vi "Add Alias_Alias.vi"(8 "error in (no error)":errorcluster, 10 "Alias Settings":T1, 11 "Aliases Ref":refnum<k24>) -> (0 "error out":errorcluster, 3 "Aliases Ref Out":refnum<k24>)   [LabVIEW 2019, in "Simple SysDef API.lvlib"]
uses:
  <userlib>/SimpleSysDef/Simple SysDef API.lvlib
  NationalInstruments.VeriStand.SystemDefinitionAPI
  <userlib>/SimpleSysDef/_SubVIs/Add Alias_Alias Settings.ctl
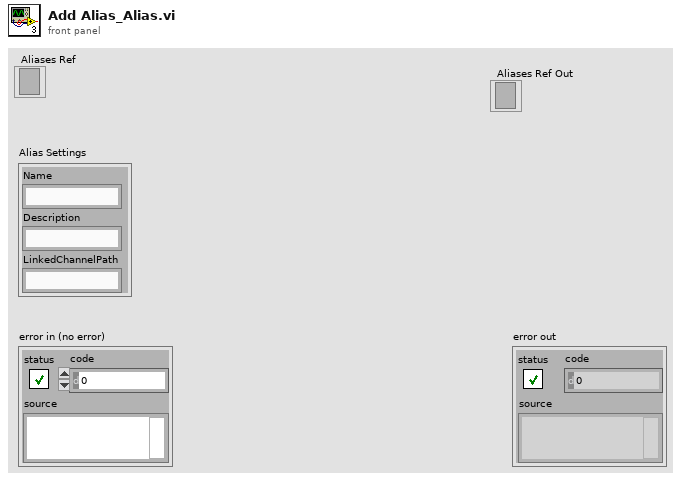
[diagram p1: front panel]
types:
  T1 = typedef "Simple SysDef API.lvlib/Add Alias_Alias Settings.ctl" = cluster{"Name":string, "Description":string, "LinkedChannelPath":string}
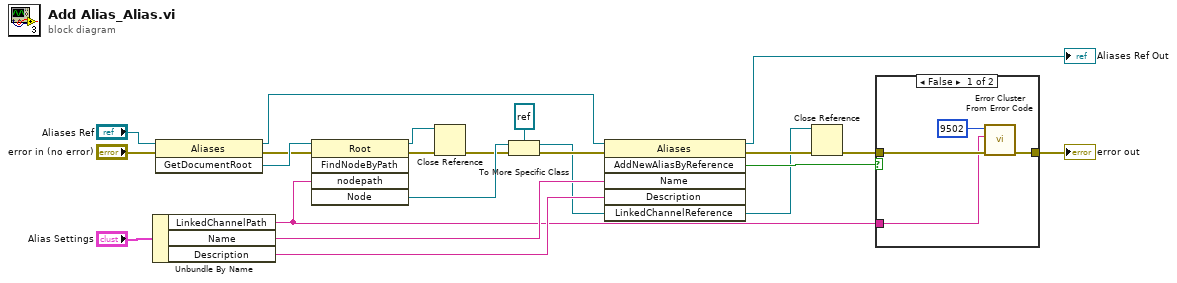
[diagram p0: block diagram]
diagram:
  n1 = Unbundle By Name("Alias Settings") -> ("LinkedChannelPath"=w9:string, "Name"=w18:string, "Description"=w16:string)
  n2 = invoke class="Aliases" method="GetDocumentRoot"(reference="Aliases Ref", error in="error in (no error)") -> (reference out=w12:refnum<k24>, error out=w11:errorcluster, "GetDocumentRoot"=w14:refnum<k24>)  [unwired: 1 in]
  n3 = invoke class="Root" method="FindNodeByPath"(reference=w14, error in=w11, "nodepath"=w9) -> (reference out=w4:refnum<k24>, error out=w10:errorcluster, "Node"=w6:refnum<k24>)  [unwired: 2 in, 2 out]
  n4 = Close Reference(reference=w4, error in (no error)=w10) -> (error out=w5:errorcluster)
  n5 = To More Specific Class(target class=refnum<k24> refnum ("LinkedChannelReference"), reference=w6, error in=w5) -> (specific class reference=w1:refnum<k24>, error out=w8:errorcluster)
  n6 = invoke class="Aliases" method="AddNewAliasByReference"(reference=w12, error in=w8, "Name"=w18, "Description"=w16, "LinkedChannelReference"=w1) -> (reference out=→"Aliases Ref Out":refnum<k24>, error out=w3:errorcluster, "AddNewAliasByReference"=w21:bool)  [unwired: 1 in, 3 out]
  n7 = Close Reference(reference=w1, error in (no error)=w3) -> (error out=w2:errorcluster)
  n8 = case shown="False" w21 {
    tunnel: w2 -> [w25 w26]
    tunnel: [w24 w26] -> w20
    tunnel: w9 -> [w22 _]
    frame False {
      n9 = call <userlib>:"Error Cluster From Error Code.vi"("error in (no error)"=w25, "error message (\"\")"=w22, "error code (0)"=9502) -> ("error out"=w24:errorcluster)  [unwired: 6 in]
    }
    frame True {
    }
  }
  "error out" <- w20
